vi "calc_logmag.vi"(11 "abs":dbl) -> (2 "power":dbl, 3 "logmag":dbl)   [LabVIEW 2025]
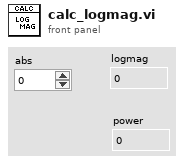
[diagram p1: front panel]
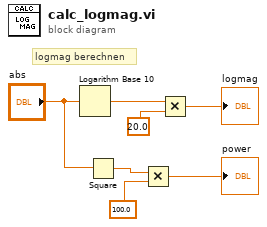
[diagram p0: block diagram]
diagram:
  # "logmag berechnen"
  n1 = Logarithm Base 10(1:"abs") -> (0:w6:dbl)
  n2 = Square(x="abs") -> (x^2=w1:dbl)
  n3 = Multiply(x=w1, y=100.0) -> (x*y=→"power":dbl)
  n4 = Multiply(x=w6, y=20.0) -> (x*y=→"logmag":dbl)
